vi "Close Server Reference.vi"(8 "error in (no error)":errorcluster, 11 "Server in":refnum<class "JSONRPC Server.lvclass">) -> (0 "error out":errorcluster)   [LabVIEW 2020, in "JSON-RPC Lib.lvlib" / "JSONRPC Server.lvclass"]
doc: "Stop the RPC Server. This uninitializes the process for all RPC Servers in this application instance."
uses:
  JSONRPC Server.lvclass
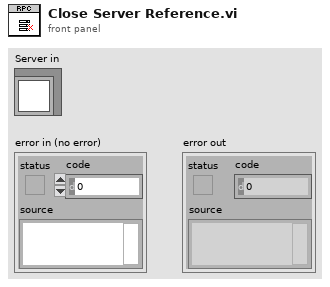
[diagram p1: front panel]
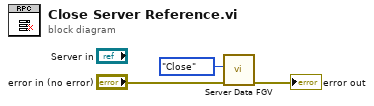
[diagram p0: block diagram]
diagram:
  n1 = call "Server Data FGV.vi"("error in (no error)"="error in (no error)", "Action"=enum16{"Initialize", "Check", "Close"}."Close") -> ("error out"=→"error out":errorcluster)  [unwired: 6 in, 3 out]
